vi "solar Refnum Type Cast (From).vi"(1 "Refnum":T1) -> (0 "SOLAR":refnum<queue>)   [LabVIEW 2018]
doc: "This type casts the solar refnum to SEQ."
uses:
  solar_ctl SOLAR Global.ctl
  solar_ctl Target Global.ctl
  voyager/solar_voy_ctl Voyager Refnum.ctl
  qtimer/solar_qtimer_ctl Refnum.ctl
  solar_ctl SOLAR Refnum.ctl
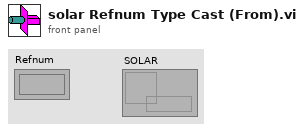
[diagram p1: front panel]
types:
  T1 = typedef "solar_ctl SOLAR Refnum.ctl" = refnum<k1>
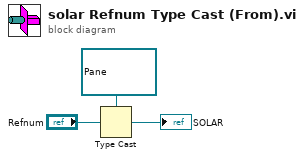
[diagram p0: block diagram]
diagram:
  n1 = Type Cast(type=refnum<queue> refnum ("SOLAR"), x="Refnum") -> (*(type *) &x=→"SOLAR":refnum<queue>)
